vi "反转判断2.vi"(6 "重置？":bool, 8 "error in (no error)":errorcluster, 9 "反转判断条件1":T1, 10 "传感器数据":dbl[](array[numeric])) -> (0 "error out":errorcluster, 2 "反转":bool)   [LabVIEW 2015, in "Action.lvlib"]
uses:
  Action.lvlib
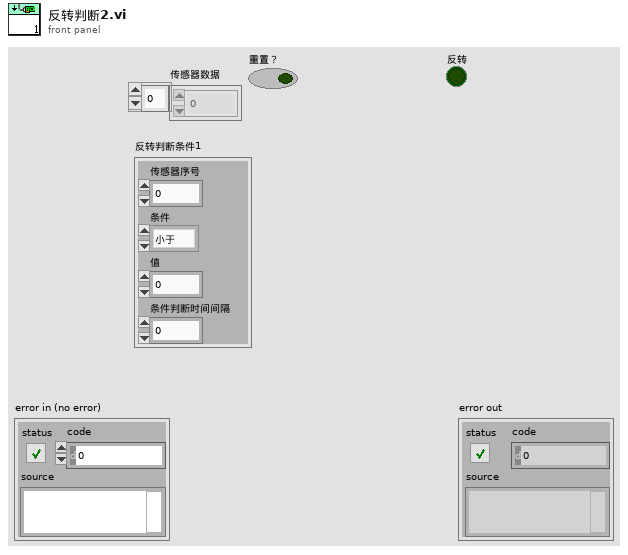
[diagram p1: front panel]
types:
  T1 = typedef "Action.lvlib/反转判断条件1.ctl" = cluster{"传感器序号":i32, "条件":enum16{"小于", "大于", "等于"}, "值":dbl, "条件判断时间间隔":i32}
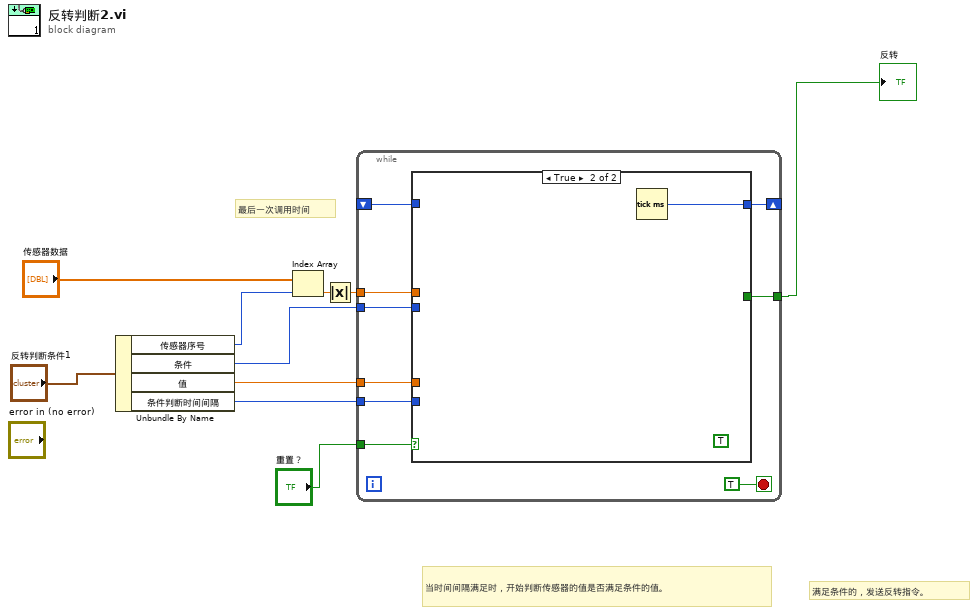
[diagram p0: block diagram]
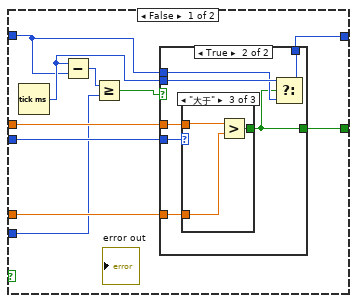
[diagram p2: hidden frame]
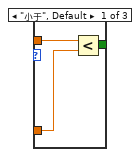
[diagram p4: hidden frame]
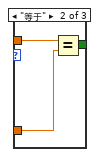
[diagram p5: hidden frame]
diagram:
  # "满足条件的，发送反转指令。"
  # "当时间间隔满足时，开始判断传感器的值是否满足条件的值。"
  # "最后一次调用时间"
  n1 = Unbundle By Name("反转判断条件1") -> ("传感器序号"=w8:i32, "条件"=w7:enum16{"小于", "大于", "等于"}, "值"=w6:dbl, "条件判断时间间隔"=w1:i32)
  n2 = Index Array(array="传感器数据", index=w8) -> (element=w4:dbl)
  n3 = Absolute Value(x=w4) -> (abs(x)=w3:dbl)
  n4 = while {
    tunnel: w7 -> [w19]
    tunnel: w3 -> [w18]
    tunnel: w6 -> [w17]
    shift-right: [w16] -> _
    shift-left: _ -> [w15]
    tunnel: w1 -> [w14]
    tunnel: [w13] -> w5
    tunnel: "重置？" -> [w11]
    stop <- TRUE stop-if-true
    n5 = case shown="True" w11 {
      tunnel: w19 -> [w29 _]
      tunnel: w18 -> [w28 _]
      tunnel: w17 -> [w27 _]
      tunnel: [w22 w47] -> w16
      tunnel: w15 -> [w23 _]
      tunnel: w14 -> [w21 _]
      tunnel: [w25 _] -> w13
      frame False {
        n6 = Tick Count (ms)() -> (millisecond timer value=w24:u32)
        n7 = Subtract(x=w24, y=w23) -> (x-y=w26:u32)
        n8 = Greater Or Equal?(x=w26, y=w21) -> (x >= y?=w20:bool)
        n9 = case shown="True" w20 {
          tunnel: w29 -> [_ w37]
          tunnel: w28 -> [_ w36]
          tunnel: w27 -> [_ w35]
          tunnel: [_ w31] -> w25
          tunnel: w24 -> [_ w34]
          tunnel: w23 -> [w30 w33]
          tunnel: [w30 w32] -> w22
          frame False {
          }
          frame True {
            n10 = case shown="\"大于\"" w37 {
              tunnel: w36 -> [w40 w43 w46]
              tunnel: w35 -> [w39 w42 w45]
              tunnel: [w38 w41 w44] -> w31
              frame "小于", Default {
                n11 = Less?(x=w40, y=w39) -> (x < y?=w38:bool)
              }
              frame "等于" {
                n12 = Equal?(x=w43, y=w42) -> (x = y?=w41:bool)
              }
              frame "大于" {
                n13 = Greater?(x=w46, y=w45) -> (0:w44:bool)
              }
            }
            n14 = Select(t=w34, s=w31, f=w33) -> (s? t:f=w32:u32)
          }
        }
      }
      frame True {
        (unwired) TRUE
        n15 = Tick Count (ms)() -> (millisecond timer value=w47:u32)
      }
    }
  }
  "反转" <- w5
